vi "Create Builder.vi"(8 "error in (no error)":errorcluster, 10 "Cluster":T1, 11 "CLI Output":refnum<class "CLI Output.lvclass">) -> (0 "error out":errorcluster, 3 "Builder out":refnum<class "Builder.lvclass">)   [LabVIEW 2019, in "Builder.lvclass"]
uses:
  Builder.lvclass
  CLI-Inputs.ctl
  TargetType.ctl
  CLI Output/CLI Output.lvclass
  Builder.lvclass/Builder.ctl
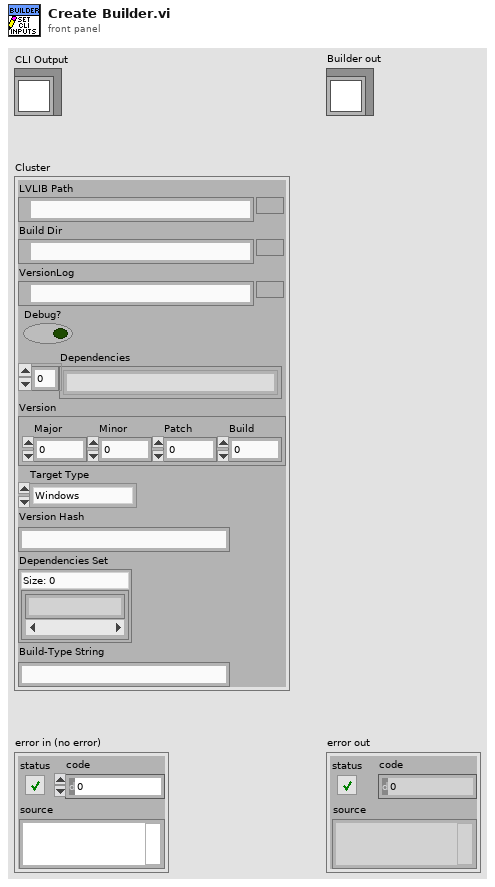
[diagram p1: front panel]
types:
  T1 = typedef "CLI-Inputs.ctl" = cluster{"LVLIB Path":path, "Build Dir":path, "VersionLog":path, "Debug?":bool, "Dependencies":string[], "Version":cluster{"Major":i32, "Minor":i32, "Patch":i32, "Build":i32}, "Target Type":T2, "Version Hash":string, "Dependencies Set":set{string}, "Build Type":string}
  T2 = typedef "TargetType.ctl" = enum16{"Windows", "cRIO-9045"}
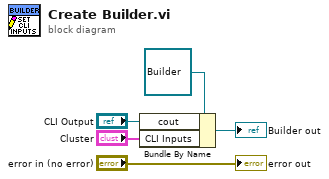
[diagram p0: block diagram]
diagram:
  n1 = Bundle By Name(cluster=refnum<class "Builder.lvclass"> refnum ("Builder.lvclass"), "cout"="CLI Output", "CLI Inputs"="Cluster") -> (→"Builder out":refnum<class "Builder.lvclass">)
  "error out" <- "error in (no error)"
